vi "Fast IV Contour V1.vi"(8 "error in":errorcluster, 11 "Book number":i32=357) -> (0 "error out":errorcluster)   [LabVIEW 2021]
uses:
  global.vi
  <vilib>/Utility/file.llb/Write Delimited Spreadsheet (DBL).vi
panel:
  in  "Tab Control":enum32{"Set IV DAQ", "Source Choice", "Scan"}(tab)=enum."Scan"
  in  "rate":dbl=100000.0 format="%#_13g"
  in  "Trigger source":tag="/Dev1/PFI12"
  in  "samples per channel":i32=2000
  in  "Voltage Read":tag="Dev1/ai1"
  in  "Vmax":dbl=2.0
  in  "Frequency Hz":dbl=50.0
  in  "Agi T or SRS F":bool=TRUE
  in  "Field uses Kei  T or DAQ F":bool=TRUE
  in  "Tab Control 2":enum32{"DAQ Field", "Kei Field"}(tab)=enum."Kei Field"
  in  "DAQ Ramp Rate V per s":dbl=0.04
  in  "DAQ Field Out Channel":i32=1
  in  "NI-DAQ Device Number":i32=1
  in  "DAQ Field Read":tag="Dev1/ai3"
  in  "Field Voltage Factor":dbl=1.0 format="%#_13g"
  in  "Init Ramp Time s":dbl=100.0
  in  "Step Ramp Time s":dbl=1.0
  in  "KEITHLEY 2400 GPIB Address":string="13"
  in  "SRS resource name":string="GPIB0::19::INSTR"
  in  "Agi Address":string="GPIB0::10::INSTR"
  in  "Start field V":dbl=-2.0 format="%#_13g"
  in  "Field step V":dbl=0.004 format="%#_13g"
  in  "End field V":dbl=2.0 format="%#_13g"
  in  "Current step uA":dbl=0.02 format="%#_13g"
  in  "Average times":i32=10
  out "Current Field mT":dbl=-7.320000000000002
  out "Current Field V":dbl=-0.7320000000000002
  in  "Field Scale factor":dbl=10.0
  in  "Return":bool=TRUE
  in  "Voltage Amp Scale factor":dbl=0.0005
  in  "Contour plot folder":path=path "C:/Users/gyue/Box Sync/Guang Yue/data/Contour plot"
  # "Field Vread x factor= Field Vapplied"
  # "Scale * Vread=Vdevice"
  # "V_Field*Scale=mT"
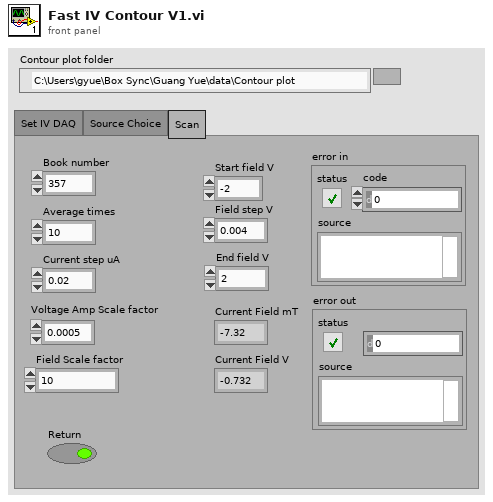
[diagram p1: front panel]
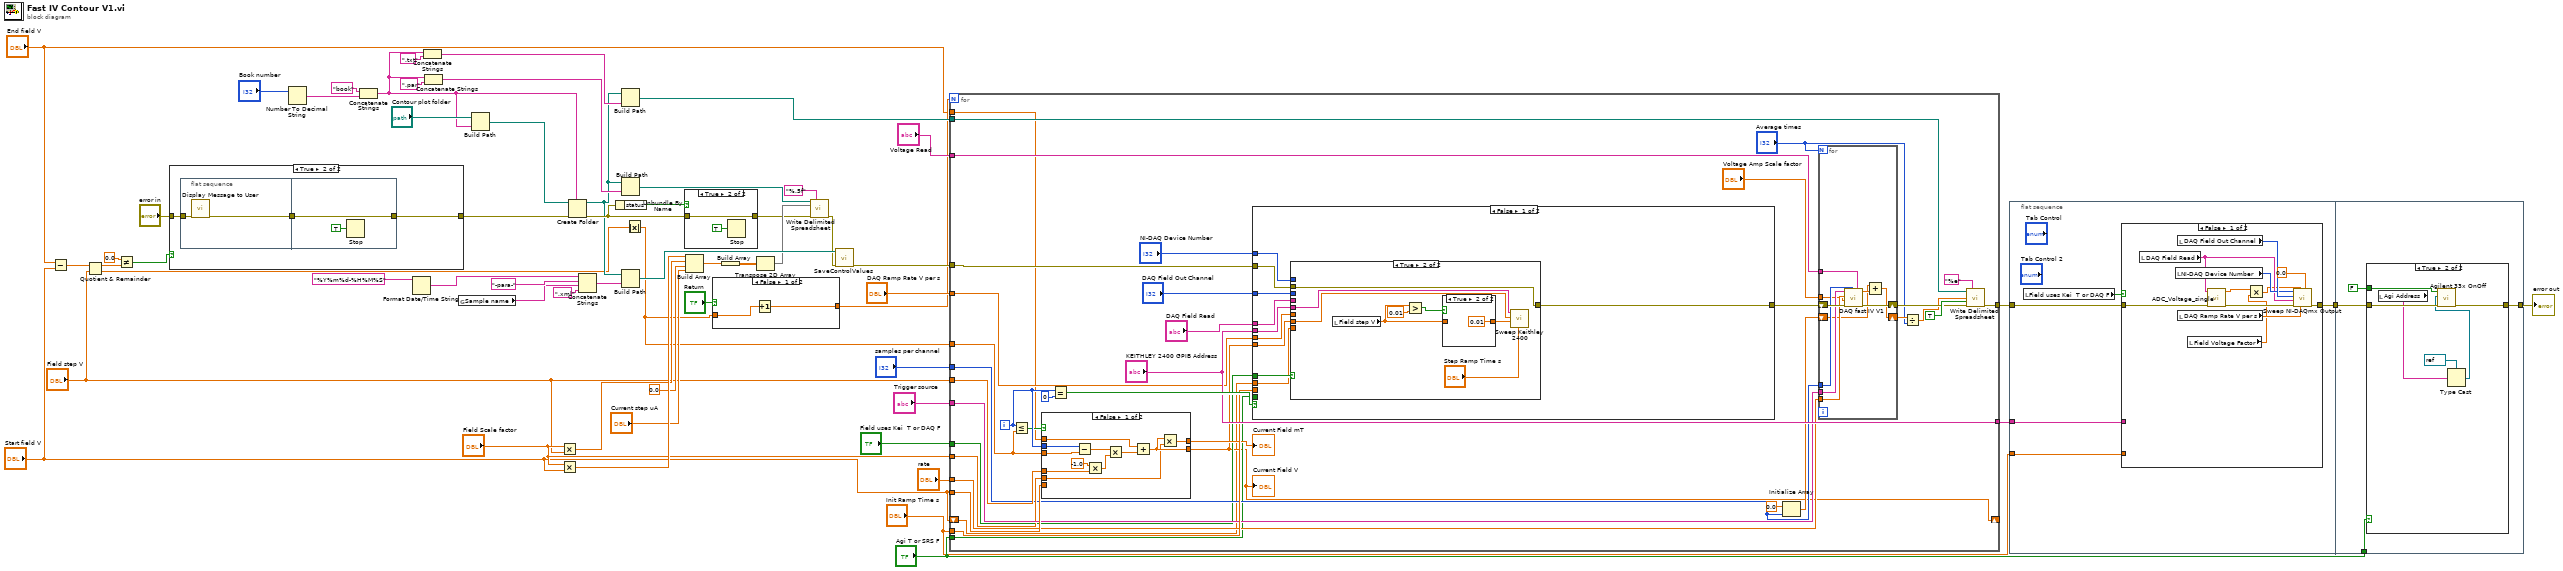
[diagram p0: block diagram]
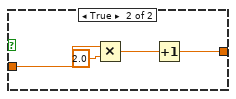
[diagram p3: hidden frame]
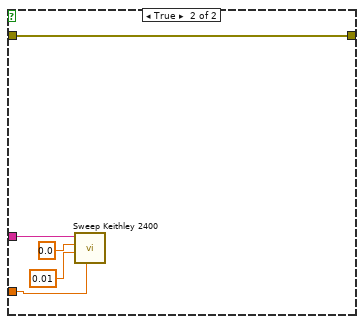
[diagram p4: hidden frame]
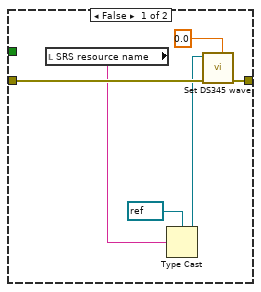
[diagram p5: hidden frame]
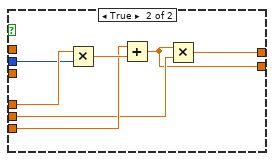
[diagram p7: hidden frame]
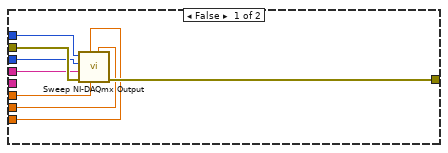
[diagram p8: hidden frame]
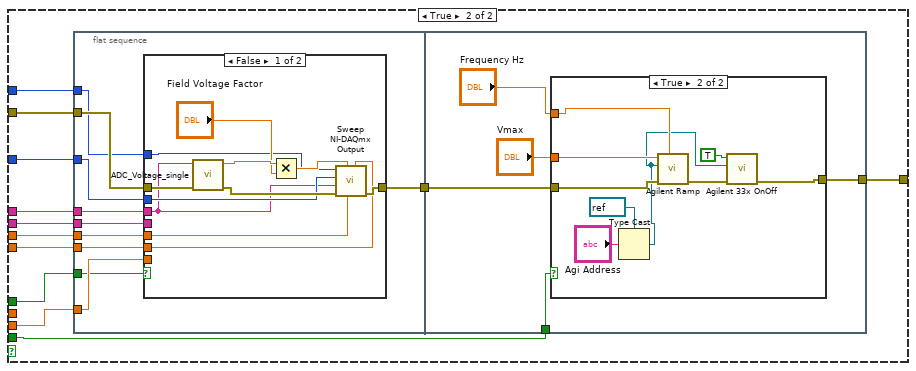
[diagram p10: hidden frame]
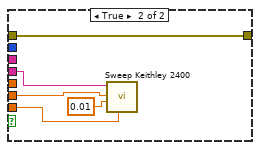
[diagram p11: hidden frame]
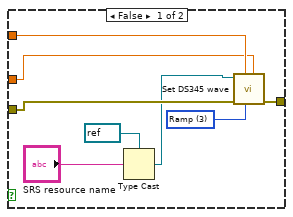
[diagram p12: hidden frame]
diagram:
  n1 = Subtract(x="End field V", y="Start field V") -> (x-y=w8:dbl)
  n2 = Quotient & Remainder(x=w8, y="Field step V") -> (x-y*floor(x/y)=w5:dbl, floor(x/y)=w6:dbl)
  n3 = Not Equal?(x=0.0, y=w5) -> (x != y?=w3:bool)
  n4 = case shown="True" w3 {
    tunnel: "error in" -> [w60 w63]
    tunnel: [w60 w61] -> w1
    frame False {
    }
    frame True {
      n5 = flat-sequence {
        tunnel: w63 -> [w65]
        tunnel: [w64] -> w62
        tunnel: w62 -> [w66]
        tunnel: [w66] -> w61
        frame #0 {
          n6 = call "Display Message to User"("error in (no error)"=w65) -> ("error out"=w64:errorcluster)  [unwired: 9 in, 1 out]
        }
        frame #1 {
          n7 = Stop(stop? (T)=TRUE) -> ()
        }
      }
    }
  }
  n8 = Number To Decimal String(number="Book number") -> (decimal integer string=w19:string)  [unwired: 1 in]
  n9 = Concatenate Strings("book" ("string"), w19) -> (w17:string)
  n10 = Format Date/Time String(time format string (%c)="%Y%m%d-%H%M%S") -> (date/time string=w37:string)  [unwired: 2 in]
  n11 = Concatenate Strings(w17, ".txt" ("string")) -> (w46:string)
  n12 = Concatenate Strings(w17, ".par" ("string")) -> (w53:string)
  n13 = global read "global.vi" "Sample name"() -> (w36:string)
  n14 = Build Path(base path="Contour plot folder", name or relative path=w17) -> (appended path=w43:path)
  n15 = Multiply(x="Field Scale factor", y="Field step V") -> (x*y=w23:dbl)
  n16 = Multiply(x="Field Scale factor", y="Start field V") -> (x*y=w25:dbl)
  n17 = Create Folder(prompt (Create Folder)=w17, path (use dialog)=w43, error in=w1) -> (created path=w38:path, error out=w40:errorcluster)  [unwired: 1 out]
  n18 = Concatenate Strings(w37, "-para-" ("string"), w36, ".xml" ("string")) -> (w57:string)
  n19 = Unbundle By Name(w40) -> ("status"=w41:bool)
  n20 = Build Path(base path=w38, name or relative path=w46) -> (appended path=w45:path)
  n21 = Build Path(base path=w38, name or relative path=w53) -> (appended path=w52:path)
  n22 = Build Path(base path=w38, name or relative path=w57) -> (appended path=w55:path)
  n23 = Absolute Value(x=w6) -> (abs(x)=w10:dbl)
  n24 = case shown="True" w41 {
    tunnel: [w68 w70] -> w39
    tunnel: w40 -> [w68 w70]
    frame False {
    }
    frame True {
      n25 = Stop(stop? (T)=TRUE) -> ()
    }
  }
  n26 = Build Array(w25, w23, 0.0 ("element"), "Current step uA") -> (w50:dbl[])
  n27 = case shown="False" "Return" {
    tunnel: w10 -> [w72 w76]
    tunnel: [w71 w73] -> w12
    frame False {
      n28 = Increment(x=w72) -> (x+1=w71:dbl)
    }
    frame True {
      n29 = Multiply(x=w76, y=2.0) -> (x*y=w74:dbl)
      n30 = Increment(x=w74) -> (x+1=w73:dbl)
    }
  }
  n31 = Build Array(w50) -> (w49:dbl[][])
  n32 = Transpose 2D Array(2D array=w49) -> (transposed array=w48:dbl[][])
  n33 = call-poly <vilib>:"Write Delimited Spreadsheet.vi"("file path (dialog if empty)"=w52, "format (%.3f)"="%.5f", "2D data"=w48, "error in (no error)"=w39) -> ("error out"=w42:errorcluster)  [unwired: 10 in, 1 out]
  n34 = call "SaveControlValues.vi"("XML File Path"=w55, "error in (no error)"=w42) -> ("error out"=w35:errorcluster)  [unwired: 8 in]
  n35 = for {
    N: w12 -> [_]
    tunnel: "Start field V" -> [w113]
    tunnel: "Field step V" -> [w112]
    tunnel: w45 -> [w108]
    tunnel: w35 -> [w106]
    tunnel: [w103] -> w34
    tunnel: ["KEITHLEY 2400 GPIB Address"] -> w33
    tunnel: "Init Ramp Time s" -> [w101]
    tunnel: "Voltage Read" -> [w99]
    tunnel: "samples per channel" -> [w91]
    tunnel: "Trigger source" -> [w98]
    tunnel: "rate" -> [w97]
    tunnel: "Field Scale factor" -> [w96]
    tunnel: "Agi T or SRS F" -> [w89]
    tunnel: "Field uses Kei  T or DAQ F" -> [w88]
    tunnel: "DAQ Ramp Rate V per s" -> [w87]
    shift-right: [w83] -> _
    shift-left: "Start field V" -> [w82]
    tunnel: w10 -> [w79]
    tunnel: "End field V" -> [w78]
    i -> [w81]
    n36 = Less Or Equal?(x=w81, y=w79) -> (x <= y?=w80:bool)
    n37 = case shown="False" w80 {
      tunnel: w113 -> [_ w130]
      tunnel: w112 -> [w120 w129]
      tunnel: w81 -> [w122 w128]
      tunnel: [w114 w127] -> w100
      tunnel: w96 -> [w115 w126]
      tunnel: [w116 w125] -> w83
      tunnel: w79 -> [w123 _]
      tunnel: w78 -> [w117 _]
      frame False {
        n38 = Subtract(x=w122, y=w123) -> (x-y=w121:dbl)
        n39 = Multiply(x=-1.0, y=w120) -> (x*y=w118:dbl)
        n40 = Multiply(x=w121, y=w118) -> (x*y=w124:dbl)
        n41 = Add(x=w117, y=w124) -> (x+y=w116:dbl)
        n42 = Multiply(x=w116, y=w115) -> (x*y=w114:dbl)
      }
      frame True {
        n43 = Multiply(x=w129, y=w128) -> (x*y=w131:dbl)
        n44 = Add(x=w130, y=w131) -> (x+y=w125:dbl)
        n45 = Multiply(x=w125, y=w126) -> (x*y=w127:dbl)
      }
    }
    "Current Field V" <- w83
    "Current Field mT" <- w100
    n46 = Equal?(x=w81, y=0) -> (x = y?=w107:bool)
    n47 = case shown="False" w107 {
      tunnel: w83 -> [w151 w176]
      tunnel: w106 -> [w148 w179]
      tunnel: [w147 w178] -> w105
      tunnel: "KEITHLEY 2400 GPIB Address" -> [w150 w181]
      tunnel: w101 -> [_ w177]
      tunnel: w89 -> [_ w175]
      tunnel: w88 -> [w149 w174]
      tunnel: w87 -> [w146 w173]
      tunnel: "DAQ Field Out Channel" -> [w144 w172]
      tunnel: "NI-DAQ Device Number" -> [w145 w171]
      tunnel: "DAQ Field Read" -> [w143 w170]
      tunnel: w82 -> [w142 _]
      frame False {
        n48 = case shown="True" w149 {
          tunnel: w151 -> [w152 w167]
          tunnel: w150 -> [_ w161]
          tunnel: w148 -> [w159 w160]
          tunnel: [w158 w160] -> w147
          tunnel: w146 -> [w157 _]
          tunnel: w145 -> [w156 _]
          tunnel: w144 -> [w155 _]
          tunnel: w143 -> [w154 _]
          tunnel: w142 -> [w153 _]
          frame False {
            n49 = call "Sweep NI-DAQmx Output.vi"("Final Output Value"=w152, "Ramp Rate V/s"=w157, "Init Input Voltage"=w153, "error in"=w159, "Field Read Voltage"=w154, "Output Channel"=w155, "NI-DAQ Device Number"=w156) -> ("error out"=w158:errorcluster)  [unwired: 4 in]
          }
          frame True {
            n50 = local read "Field step V"() -> (w162:dbl)
            n51 = Greater?(x=w162, y=0.01) -> (0:w164:bool)
            n52 = case shown="True" w164 {
              tunnel: [w168 0.01 ("Gate Step [V]")] -> w163
              tunnel: w162 -> [w168 _]
              frame False {
              }
              frame True {
              }
            }
            n53 = call "Sweep Keithley 2400.vi"("Ramp Time (s)"="Step Ramp Time s", "Gate Step [V]"=w163, "final gate voltage (V)"=w167, "KEITHLEY 2400 GPIB Address"=w161) -> ()  [unwired: 6 in, 2 out]
          }
        }
      }
      frame True {
        n54 = flat-sequence {
          tunnel: w176 -> [w191]
          tunnel: w181 -> [w190]
          tunnel: [w186] -> w180
          tunnel: w179 -> [w187]
          tunnel: w177 -> [w189]
          tunnel: w174 -> [w188]
          tunnel: w173 -> [w185]
          tunnel: w172 -> [w184]
          tunnel: w171 -> [w183]
          tunnel: w170 -> [w182]
          tunnel: w180 -> [w212]
          tunnel: [w211] -> w178
          tunnel: w175 -> [w208]
          frame #0 {
            n55 = case shown="False" w188 {
              tunnel: w191 -> [w196 w207]
              tunnel: w190 -> [_ w206]
              tunnel: w189 -> [_ w205]
              tunnel: w187 -> [w198 w203]
              tunnel: [w197 w203] -> w186
              tunnel: w185 -> [w195 _]
              tunnel: w184 -> [w194 _]
              tunnel: w183 -> [w193 _]
              tunnel: w182 -> [w192 _]
              frame False {
                n56 = call "ADC_Voltage_single.vi"("error in"=w198, "physical channels"=w192) -> ("error out"=w202:errorcluster, "data"=w201:dbl)  [unwired: 8 in]
                n57 = Multiply(x=w201, y="Field Voltage Factor") -> (x*y=w199:dbl)
                n58 = call "Sweep NI-DAQmx Output.vi"("Final Output Value"=w196, "Ramp Rate V/s"=w195, "Init Input Voltage"=w199, "error in"=w202, "Field Read Voltage"=w192, "Output Channel"=w194, "NI-DAQ Device Number"=w193) -> ("error out"=w197:errorcluster)  [unwired: 4 in]
              }
              frame True {
                n59 = call "Sweep Keithley 2400.vi"("Ramp Time (s)"=w205, "Gate Step [V]"=0.01, "final gate voltage (V)"=w207, "KEITHLEY 2400 GPIB Address"=w206) -> ()  [unwired: 6 in, 2 out]
              }
            }
          }
          frame #1 {
            n60 = case shown="True" w208 {
              tunnel: w212 -> [w220 w229]
              tunnel: [w219 w227] -> w211
              tunnel: "Vmax" -> [w216 w225]
              tunnel: "Frequency Hz" -> [w217 w224]
              frame False {
                w218 = u16 3 items=["Sine", "Square", "Triangle", "Ramp", "Noise"] ("Waveform Function (0: Sine)")
                n61 = Type Cast(type=refnum<visa-resource-name> refnum ("SRS resource name 2"), x="SRS resource name") -> (*(type *) &x=w213:refnum<visa-resource-name>)
                n62 = call "Set DS345 wave.vi"("Amplitude (0.01 Vpp)"=w216, "Waveform Function (0: Sine)"=w218, "Frequency (1000 Hz)"=w217, "error in (no error)"=w220, "VISA resource name"=w213) -> ("error out"=w219:errorcluster)  [unwired: 6 in]
              }
              frame True {
                n63 = Type Cast(type=refnum<visa-resource-name> refnum ("SRS resource name 2"), x="Agi Address") -> (*(type *) &x=w221:refnum<visa-resource-name>)
                n64 = call "Agilent Ramp.vi"("Frequency Hz"=w224, "error in (no error)"=w229, "VISA resource name"=w221, "Vmax"=w225) -> ("error out"=w228:errorcluster)  [unwired: 7 in]
                n65 = call "Agilent 33x OnOff.vi"("error in (no error)"=w228, "VISA resource name"=w221, "Enable Output  (T: Enable)"=TRUE) -> ("error out"=w227:errorcluster)  [unwired: 8 in]
              }
            }
          }
        }
      }
    }
    n66 = Initialize Array(0.0 ("element"), w91) -> (w90:dbl[])
    n67 = for {
      N: "Average times" -> [_]
      tunnel: w99 -> [w139]
      tunnel: w91 -> [w138]
      tunnel: w98 -> [w137]
      tunnel: w97 -> [w136]
      shift-right: [w140] -> w104
      shift-left: w105 -> [w141]
      shift-right: [w134] -> w95
      shift-left: w90 -> [w133]
      tunnel: "Voltage Amp Scale factor" -> [w132]
      n68 = call "DAQ fast IV V1.vi"("physical channels"=w139, "samples per channel"=w138, "error in"=w141, "Scale factor"=w132, "rate"=w136, "Trigger source"=w137) -> ("error out"=w140:errorcluster, "data"=w135:dbl[])  [unwired: 4 in]
      n69 = Add(x=w133, y=w135) -> (x+y=w134:dbl[])
    }
    n70 = Divide(x=w95, y="Average times") -> (x/y=w93:dbl[])
    n71 = call-poly <vilib>:"Write Delimited Spreadsheet.vi"("file path (dialog if empty)"=w108, "format (%.3f)"="%e", "1D data"=w93, "append to file? (new file:F)"=TRUE ("append to file? (F)"), "error in (no error)"=w104) -> ("error out"=w103:errorcluster)  [unwired: 9 in, 1 out]
  }
  n72 = flat-sequence {
    tunnel: w34 -> [w231]
    tunnel: w33 -> [w234]
    tunnel: [w230] -> w31
    tunnel: "Init Ramp Time s" -> [w233]
    tunnel: [w253] -> w32
    tunnel: w31 -> [w254]
    tunnel: "Agi T or SRS F" -> [w251]
    frame #0 {
      n73 = local read "Field uses Kei  T or DAQ F"() -> (w232:bool)
      n74 = case shown="False" w232 {
        tunnel: w234 -> [_ w249]
        tunnel: w233 -> [_ w248]
        tunnel: w231 -> [w237 w246]
        tunnel: [w236 w246] -> w230
        frame False {
          n75 = local read "DAQ Field Read"() -> (w242:tag)
          n76 = local read "NI-DAQ Device Number"() -> (w243:i32)
          n77 = local read "DAQ Field Out Channel"() -> (w244:i32)
          n78 = local read "DAQ Ramp Rate V per s"() -> (w245:dbl)
          n79 = local read "Field Voltage Factor"() -> (w235:dbl)
          n80 = call "ADC_Voltage_single.vi"("error in"=w237, "physical channels"=w242) -> ("error out"=w239:errorcluster, "data"=w240:dbl)  [unwired: 8 in]
          n81 = Multiply(x=w240, y=w235) -> (x*y=w241:dbl)
          n82 = call "Sweep NI-DAQmx Output.vi"("Final Output Value"=0.0, "Ramp Rate V/s"=w245, "Init Input Voltage"=w241, "error in"=w239, "Field Read Voltage"=w242, "Output Channel"=w244, "NI-DAQ Device Number"=w243) -> ("error out"=w236:errorcluster)  [unwired: 4 in]
        }
        frame True {
          n83 = call "Sweep Keithley 2400.vi"("Ramp Time (s)"=w248, "Gate Step [V]"=0.01, "final gate voltage (V)"=0.0, "KEITHLEY 2400 GPIB Address"=w249) -> ()  [unwired: 6 in, 2 out]
        }
      }
    }
    frame #1 {
      n84 = case shown="True" w251 {
        tunnel: w254 -> [w260 w266]
        tunnel: [w259 w265] -> w253
        tunnel: FALSE ("Enable Output  (T: Enable)") -> [_ w264]
        frame False {
          n85 = local read "SRS resource name"() -> (w255:string)
          n86 = Type Cast(type=refnum<visa-resource-name> refnum ("SRS resource name 2"), x=w255) -> (*(type *) &x=w256:refnum<visa-resource-name>)
          n87 = call "Set DS345 wave.vi"("Amplitude (0.01 Vpp)"=0.0, "error in (no error)"=w260, "VISA resource name"=w256) -> ("error out"=w259:errorcluster)  [unwired: 8 in]
        }
        frame True {
          n88 = local read "Agi Address"() -> (w262:string)
          n89 = Type Cast(type=refnum<visa-resource-name> refnum ("SRS resource name 2"), x=w262) -> (*(type *) &x=w261:refnum<visa-resource-name>)
          n90 = call "Agilent 33x OnOff.vi"("error in (no error)"=w266, "VISA resource name"=w261, "Enable Output  (T: Enable)"=w264) -> ("error out"=w265:errorcluster)  [unwired: 8 in]
        }
      }
    }
  }
  "error out" <- w32
